vi "parse buttons.vi"(8 "error in (no error)":errorcluster, 11 "control\ncluster":T2) -> (0 "error out":errorcluster, 3 "control\ncluster out":T2)   [LabVIEW 2023]
uses:
  ctrl defs/ctrl controllers.ctl
  ctrl defs/ctrl Logitech Extreme 3D Pro-buttons.ctl
  ctrl defs/ctrl FRONT FACE selector.ctl
  Global odometry.vi
  ctrl defs/ctrl DRIVING FRAME selector.ctl
panel:
  in  "button for\nCG PIVOT":T1=enum."btn #12"
  in  "button for\nGEOM CTR PIVOT":T1=enum."btn #11"
  in  "button for\nAPRIL TAGS":T1=enum."btn #5"
  in  "button for\nfront/rear\ndrive direction":T1=enum."btn #6"
  in  "button for\nROBO/FLD\ncentric drive":T1=enum."btn #7"
  out "Buttons":bool[](array[boolean])
  out "POVs":i16[](array[numeric])
  out "Axes":dbl[](array[numeric])
  in  "notes":string="Joystick 0 - pilot\n\ntoggle between robo-centric and field-centric driving\n\ntoggle between front (intake) and rear (shooter) sides\n\ntoggle APRIL TAGS\n\nNOTE: labels on joystick are labeled 1-12 but programmed 0-11"
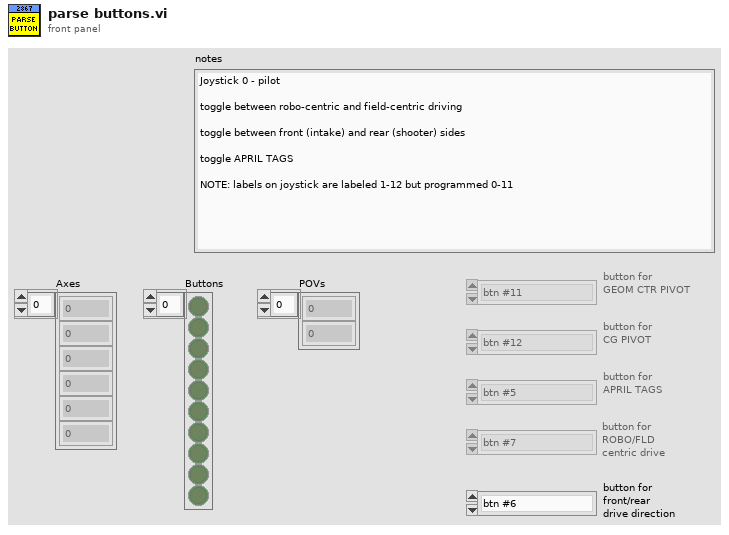
[diagram p1: front panel]
types:
  T1 = typedef "ctrl Logitech Extreme 3D Pro-buttons.ctl" = enum16{"trigger", "left-side thumb", "btn #3", "btn #4", "btn #5", "btn #6", "btn #7", "btn #8", "btn #9", "btn #10", "btn #11", "btn #12"}
  T2 = typedef "ctrl controllers.ctl" = cluster{"Axes":dbl[], "Buttons":bool[], "POVs":i16[]}
  T3 = typedef "ctrl FRONT FACE selector.ctl" = enum16{"intake side", "shooter side"}
  T4 = typedef "ctrl DRIVING FRAME selector.ctl" = enum16{"ROBO-centric", "FLD-centric"}
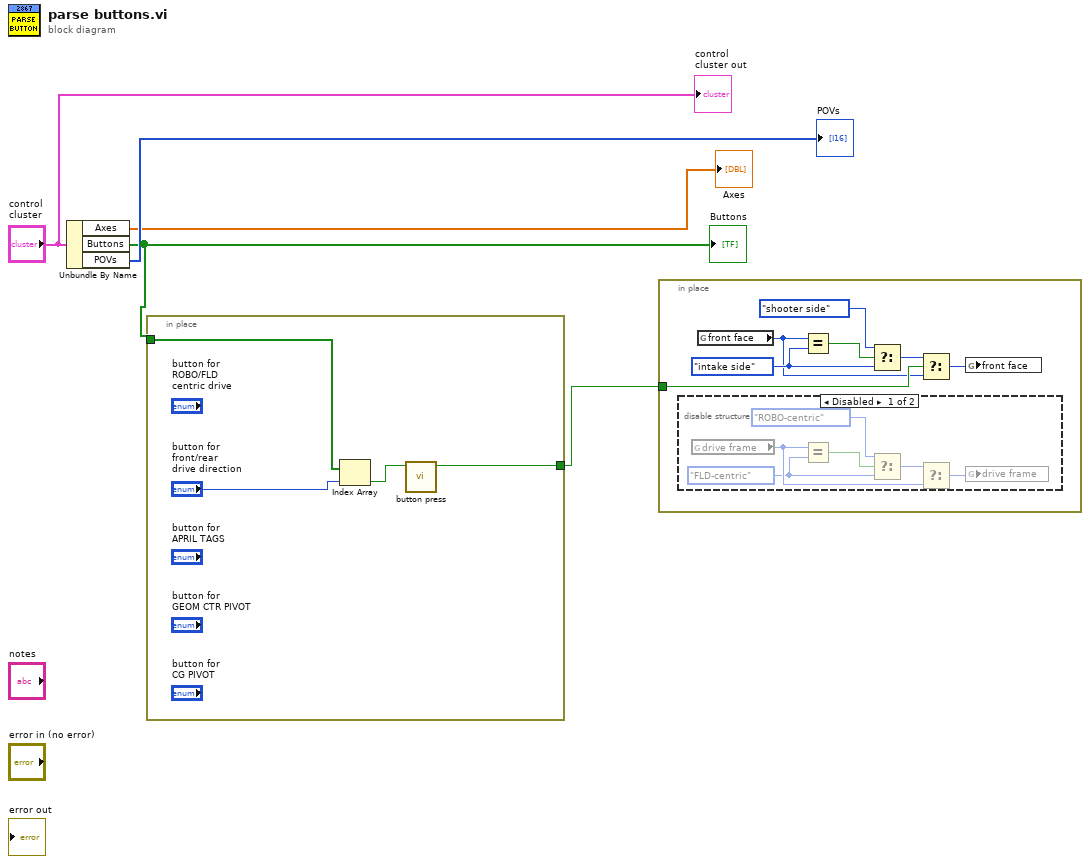
[diagram p0: block diagram]
diagram:
  n1 = Unbundle By Name("control\ncluster") -> ("Axes"=→"Axes":dbl[], "Buttons"=w2:bool[], "POVs"=→"POVs":i16[])
  "Buttons" <- w2
  n2 = in-place {
    in-place-border: w2 -> [w9]
    in-place-border: [w8] -> w4
    n3 = Index Array(array=w9, index="button for\nfront/rear\ndrive direction") -> (element=w7:bool)
    n4 = call "button press.vi"("button IN"=w7) -> ("Button Pressed?"=w8:bool)  [unwired: 10 in]
  }
  n5 = in-place {
    in-place-border: w4 -> [w15]
    w13 = ctrl_FRONT_FACE_selector."intake side" ("front face")
    n6 = disable-structure shown="Disabled" {
      frame Disabled {
        w17 = ctrl_DRIVING_FRAME_selector."FLD-centric" ("drive frame")
        n7 = global read "Global odometry.vi" "drive frame"() -> (w21:T4)
        n8 = Equal?(x=w21, y=w17) -> (x = y?=w20:bool)
        n9 = Select(t=ctrl_DRIVING_FRAME_selector."ROBO-centric" ("drive frame"), s=w20, f=w17) -> (s? t:f=w18:T4)
        n10 = Select(t=w18, f=w21) -> (s? t:f=w22:T4)  [unwired: 1 in]
        n11 = global write "Global odometry.vi" "drive frame"(w22) -> ()
      }
      frame Enabled {
      }
    }
    n12 = global read "Global odometry.vi" "front face"() -> (w11:T3)
    n13 = Equal?(x=w11, y=w13) -> (x = y?=w14:bool)
    n14 = Select(t=ctrl_FRONT_FACE_selector."shooter side" ("front face"), s=w14, f=w13) -> (s? t:f=w10:T3)
    n15 = Select(t=w10, s=w15, f=w11) -> (s? t:f=w16:T3)
    n16 = global write "Global odometry.vi" "front face"(w16) -> ()
  }
  "control\ncluster out" <- "control\ncluster"
